vi "Delete Insert Test.vi"() -> ()   [LabVIEW 2017]
uses:
  JSONtext.lvlib
  <vilib>/addons/_JKI Toolkits/Caraya/classes/Test/Test.lvclass
  <vilib>/addons/_JKI Toolkits/Caraya/classes/Assert/Assert.lvclass
panel:
  out "error out":errorcluster
  out "Array 2":string[](array[string])
  out "Passed":bool[](array[boolean])
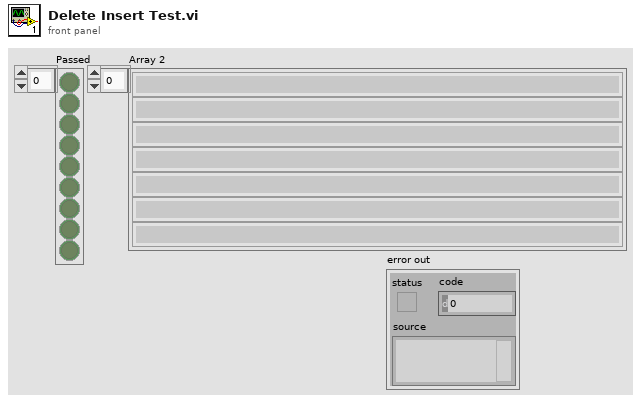
[diagram p1: front panel]
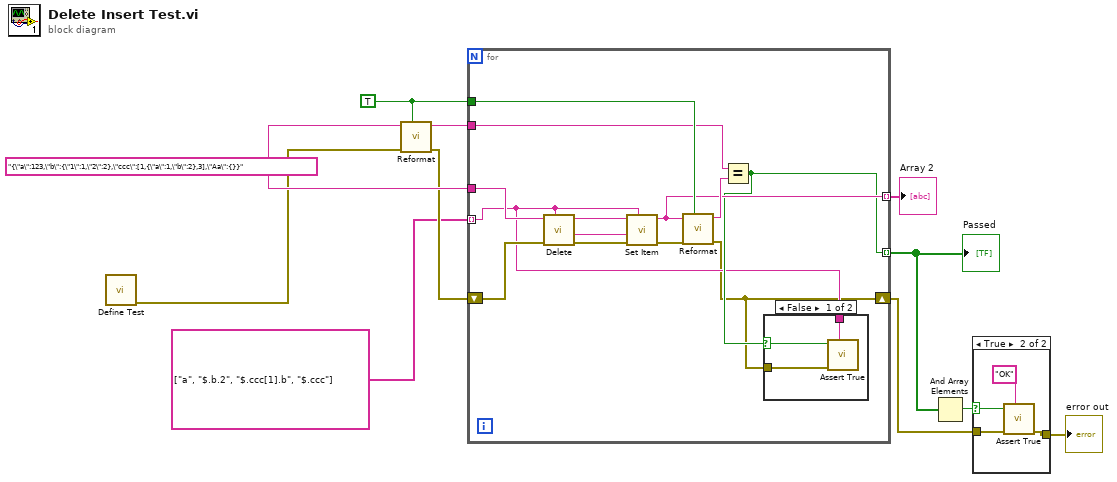
[diagram p0: block diagram]
diagram:
  w10 = TRUE ("Alphabetical Sort Objects")
  w11 = "{\"a\":123,\"b\":{\"1\":1,\"2\":2},\"ccc\":[1,{\"a\":1,\"b\":2},3],\"Aa\":{}}"
  n1 = call <vilib>:"Define Test.vi"() -> ("error out"=w4:errorcluster)  [unwired: 11 in]
  n2 = call "Reformat.vi"("Alphabetically Sort Objects"=w10, "error in (no error)"=w4, "JSON"=w11) -> ("error out"=w3:errorcluster, "<JSON>First JSON Value\n\n<JSON>"=w9:string)  [unwired: 5 in, 2 out]
  n3 = for {
    tunnel: w11 -> [w23]
    tunnel: string[] ["a", "$.b.2", "$.ccc[1].b", "$.ccc"] ("Item Names") -> [w13] mode=indexing
    tunnel: [w14] -> w6 mode=indexing
    tunnel: w10 -> [w20]
    tunnel: w9 -> [w18]
    tunnel: [w17] -> w8 mode=indexing
    shift-right: [w12] -> w5
    shift-left: w3 -> [w15]
    n4 = call "Delete.vi"("$Path or Item Name"=w13, "error in (no error)"=w15, "JSON"=w23) -> ("error out"=w16:errorcluster, "<JSON> First Deleted Item"=w22:string, "<JSON>"=w24:string)  [unwired: 4 in, 1 out]
    n5 = call "Set Item.vi"("$Path or Item Name"=w13, "error in (no error)"=w16, "JSON to Insert"=w22, "JSON"=w24) -> ("error out"=w21:errorcluster, "<JSON>"=w17:string)  [unwired: 4 in, 1 out]
    n6 = call "Reformat.vi"("Alphabetically Sort Objects"=w20, "error in (no error)"=w21, "JSON"=w17) -> ("error out"=w12:errorcluster, "<JSON>First JSON Value\n\n<JSON>"=w19:string)  [unwired: 5 in, 2 out]
    n7 = Equal?(x=w18, y=w19) -> (x = y?=w14:bool)
    n8 = case shown="False" w14 {
      selector: w14 -> [w27 _]
      tunnel: w13 -> [w26 _]
      tunnel: w12 -> [w25 _]
      frame False {
        n9 = call <vilib>:"Assert True.vi"("Label"=w26, "error in (no error)"=w25, "True?"=w27) -> ()  [unwired: 8 in, 1 out]
      }
      frame True {
      }
    }
  }
  "Passed" <- w6
  "Array 2" <- w8
  n10 = And Array Elements(Boolean array=w6) -> (logical AND=w7:bool)
  n11 = case shown="True" w7 {
    selector: w7 -> [_ w32]
    tunnel: w5 -> [w28 w30]
    tunnel: [w28 w29] -> w2
    frame False {
    }
    frame True {
      n12 = call <vilib>:"Assert True.vi"("Label"="OK", "error in (no error)"=w30, "True?"=w32) -> ("error out"=w29:errorcluster)  [unwired: 8 in]
    }
  }
  "error out" <- w2
